vi "ElapsedTimeSubVI.vi"() -> (3 "Elapsed Time (s)":dbl)   [LabVIEW 2019]
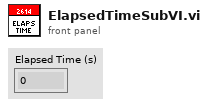
[diagram p1: front panel]
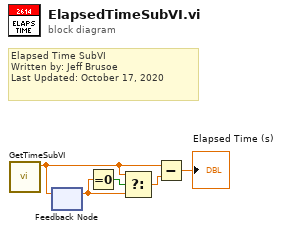
[diagram p0: block diagram]
diagram:
  # "Elapsed Time SubVI\nWritten by: Jeff Brusoe\nLast Updated: October 17, 2020"
  n1 = call "GetTimeSubVI.vi"() -> ("Seconds"=w1:dbl)  [unwired: 11 in]
  n2 = feedback-in #1(w1) -> ()
  n3 = feedback #1() -> (w3:dbl)  [unwired: 1 in]
  n4 = Equal To 0?(x=w3) -> (x = 0?=w4:bool)
  n5 = Select(t=w1, s=w4, f=w3) -> (s? t:f=w2:dbl)
  n6 = Subtract(x=w1, y=w2) -> (x-y=→"Elapsed Time (s)":dbl)
